vi "Subvi oscillator.vi"(10 "Input":bool) -> (2 "Output":bool)   [LabVIEW 2017]
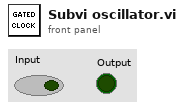
[diagram p1: front panel]
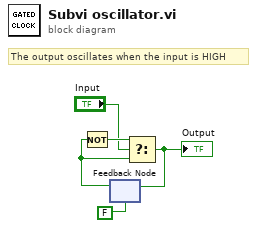
[diagram p0: block diagram]
diagram:
  # "The output oscillates when the input is HIGH"
  n1 = feedback #1(FALSE) -> (w1:bool)
  n2 = Not(x=w1) -> (.not. x?=w4:bool)
  n3 = Select(t=w4, s="Input", f=w1) -> (s? t:f=w2:bool)
  "Output" <- w2
  n4 = feedback-in #1(w2) -> ()
